vi "Transpose array.vi"(11 "BD Count":string[](array[string])) -> (3 "Array":string[][](array[string]))   [LabVIEW 2017]
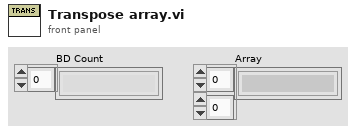
[diagram p1: front panel]
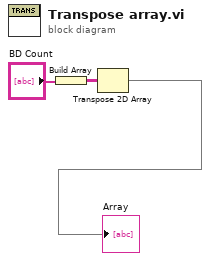
[diagram p0: block diagram]
diagram:
  n1 = Build Array("BD Count") -> (w1:string[][])
  n2 = Transpose 2D Array(2D array=w1) -> (transposed array=→"Array":string[][])
